vi "GetBDTerminals.vi"(5 "Diagram":refnum<class "Diagram.lvclass">, 6 "error in":errorcluster, 9 "VI Interpreter in":refnum<class "VI Interpreter.lvclass">) -> (0 "error out":errorcluster, 3 "VI Interpreter out":refnum<class "VI Interpreter.lvclass">, 4 "Diagram out":refnum<class "Diagram.lvclass">)   [LabVIEW 2014, in "VI Interpreter.lvclass"]
uses:
  VI Interpreter.lvclass
  Diagram/Diagram.lvclass
  Diagram/Diagram.lvclass/Diagram.ctl
  ControlTerminal/ControlTerminal.lvclass
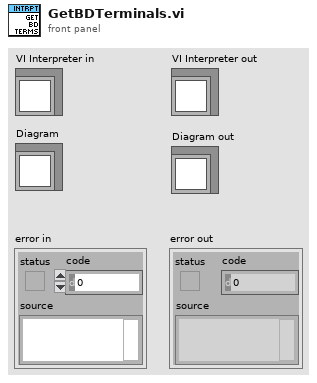
[diagram p1: front panel]
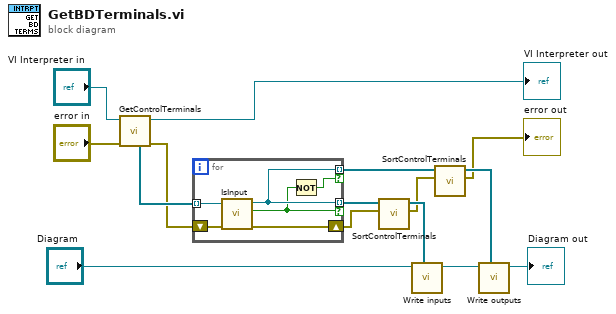
[diagram p0: block diagram]
diagram:
  n1 = call "GetControlTerminals.vi"("error in"="error in", "VI Interpreter in"="VI Interpreter in") -> ("error out"=w11:errorcluster, "VI Interpreter out"=→"VI Interpreter out":refnum<class "VI Interpreter.lvclass">, "controls"=w12:refnum<class "ControlTerminal.lvclass">[])  [unwired: 5 in]
  n2 = for {
    tunnel: w12 -> [w21] mode=indexing
    tunnel: [w20] -> w5 mode=indexing if=w18
    tunnel: [w20] -> w7 mode=indexing if=w19
    shift-right: [w16] -> w1
    shift-left: w11 -> [w17]
    n3 = call-dynamic "IsInput.vi"("error in"=w17, "ControlTerminal in"=w21) -> ("error out"=w16:errorcluster, "input"=w18:bool, "ControlTerminal out"=w20:refnum<class "ControlTerminal.lvclass">)  [unwired: 5 in]
    n4 = Not(x=w18) -> (.not. x?=w19:bool)
  }
  n5 = call "SortControlTerminals.vi"("error in"=w1, "ControlTerminals in"=w5) -> ("error out"=w3:errorcluster, "ControlTerminals out"=w4:refnum<class "ControlTerminal.lvclass">[])  [unwired: 8 in]
  n6 = call "Write inputs.vi"("inputs"=w4, "Diagram in"="Diagram") -> ("Diagram out"=w9:refnum<class "Diagram.lvclass">)  [unwired: 7 in]
  n7 = call "SortControlTerminals.vi"("error in"=w3, "ControlTerminals in"=w7) -> ("error out"=→"error out":errorcluster, "ControlTerminals out"=w6:refnum<class "ControlTerminal.lvclass">[])  [unwired: 8 in]
  n8 = call "Write outputs.vi"("outputs"=w6, "Diagram in"=w9) -> ("Diagram out"=→"Diagram out":refnum<class "Diagram.lvclass">)  [unwired: 7 in]
